vi "Main_XYA.vi"() -> ()   [LabVIEW 2024]
panel:
  in  "Use Puzzle":bool
  out "Answer":u32
  in  "Puzzle":string
  in  "Example":string
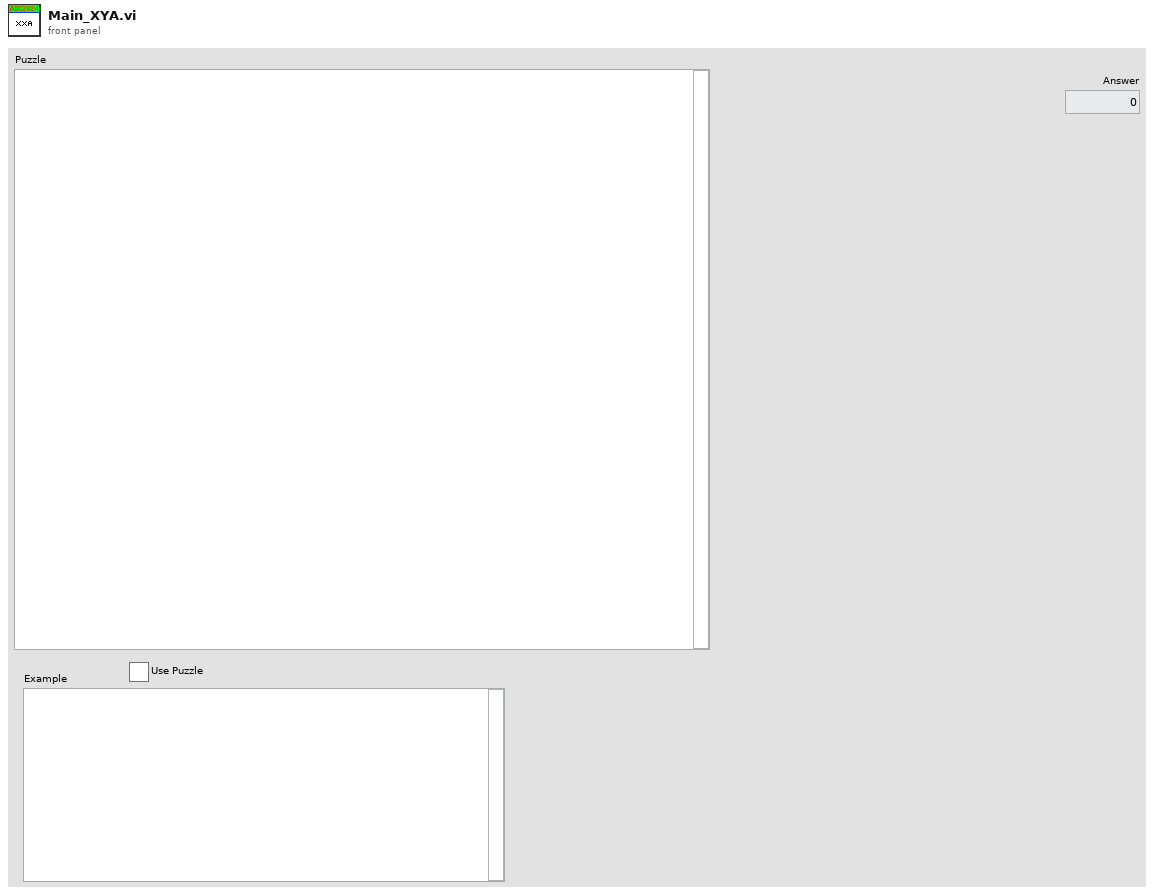
[diagram p1: front panel]
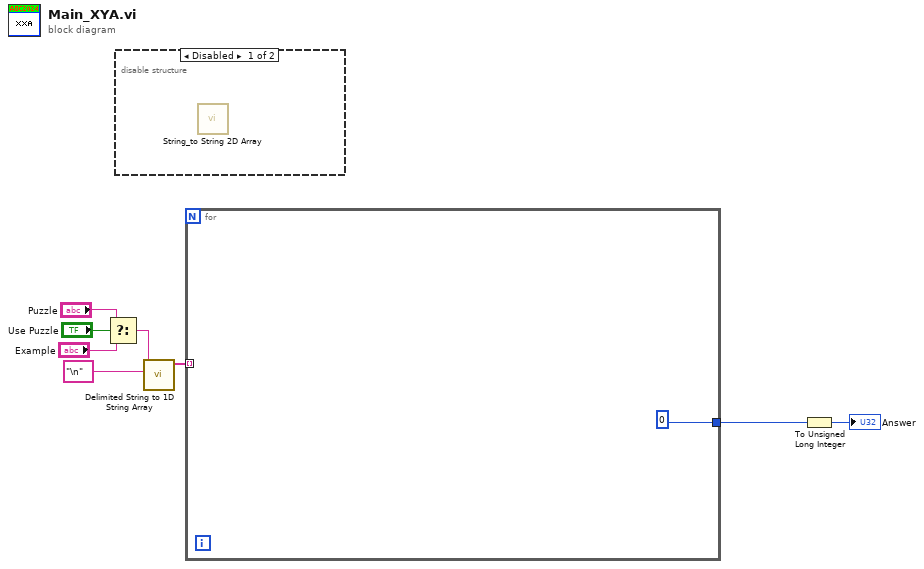
[diagram p0: block diagram]
diagram:
  n1 = Select(t="Puzzle", s="Use Puzzle", f="Example") -> (s? t:f=w3:string)
  n2 = disable-structure shown="Disabled" {
    frame Disabled {
      n3 = call "String_to String 2D Array.vi"() -> ()  [unwired: 11 in, 1 out]
    }
    frame Enabled {
    }
  }
  n4 = call <vilib>:"Delimited String to 1D String Array.vi"("delimiter"="\n" ("delimiter (Tab)"), "delimited string"=w3) -> ("string array"=w7:string[])  [unwired: 9 in]
  n5 = for {
    tunnel: w7 -> [_] mode=indexing
    tunnel: [0] -> w5
  }
  n6 = To Unsigned Long Integer(number=w5) -> (unsigned 32bit integer=→"Answer":u32)
